vi "Move_Twin_Stacks.vi"(3 "Mode":T5, 5 "Traverse line In":T2 {"Row Duration (mins)" format="%#.1f"; "Row No" min=0; "Trace Gas Concentration (%)" min=0.0 format="%#.2f"; "Emission Rate (l/min)" format="%#.2f"; "Tunnel Speed" format="%#.2f"; "Start X" format="%#.2f"; "Start Y" format="%#.2f"; "Start Z" format="%#.2f"; "End X" format="%#.2f"; "End Y" format="%#.2f"; "End Z" format="%#.2f"; "Averaging time (min)" min=0.0 format="%#.2f"}) -> (0 "Error Message":string, 1 "Status":T1, 2 "Traverse line Out":T2 {"Row Duration (mins)" format="%#.1f"; "Row No" min=0; "Trace Gas Concentration (%)" min=0.0 format="%#.2f"; "Emission Rate (l/min)" format="%#.2f"; "Tunnel Speed" format="%#.2f"; "Start X" format="%#.2f"; "Start Y" format="%#.2f"; "Start Z" format="%#.2f"; "End X" format="%#.2f"; "End Y" format="%#.2f"; "End Z" format="%#.2f"; "Averaging time (min)" min=0.0 format="%#.2f"})   [LabVIEW 2010]
uses:
  Gen Trav/Traverse_cluster.ctl
  Gen Trav/Spacing.ctl
  Controls/Multi_run_mode.ctl
  Controls/User_Specific_mode.ctl
  Gen Trav/Multi_Run_Status.ctl
  ADAM Client/Sub VIs/ADAM Controls/Update_scan_value.ctl
panel:
  out "Delta X":dbl
  out "Trav Position":dbl
  out "Dumb Position":dbl
  # "X           Y            Z"
  # "Start"
  # "End"
  # "X           Y            Z"
  # "Start"
  # "End"
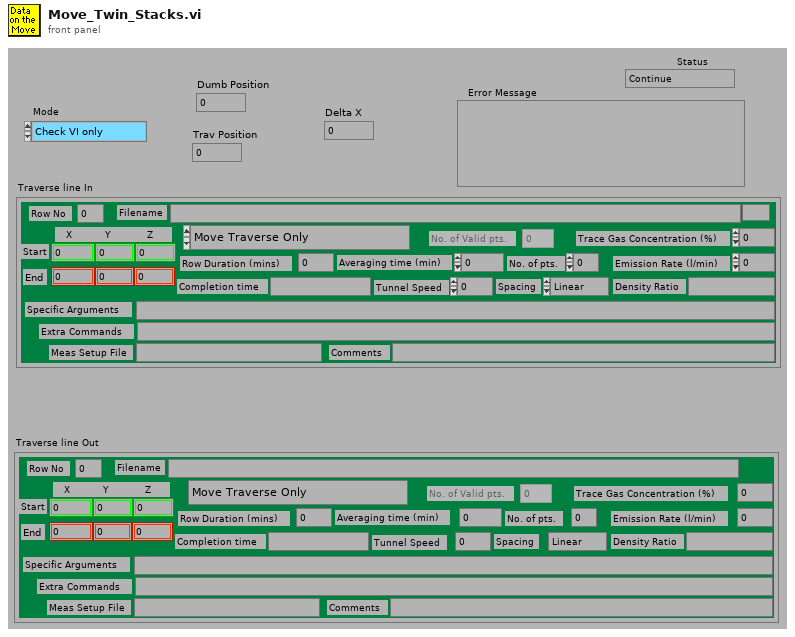
[diagram p1: front panel]
types:
  T1 = typedef "Multi_Run_Status.ctl" = enum16{"Continue", "Jump to Next Point", "Jump to Next Row", "Jump To Fall Back", "Terminate Run"}
  T2 = typedef "Traverse_cluster.ctl" = cluster{"Start X":dbl, "Start Y":dbl, "Start Z":dbl, "End X":dbl, "End Y":dbl, "End Z":dbl, "No. of pts.":i32, "Spacing":T3, "Filename":path, "Tunnel Speed":dbl, "Averaging time (min)":dbl, "Extra Commands":string, "Specific Arguments":string, "Emission Rate (l/min)":dbl, "Trace Gas Concentration (%)":dbl, "Density Ratio":string, "Comments":string, "Row No":i32, "Row Type Selector":T4, "Completion time":string, "Row Duration (mins)":dbl, "No. of Valid pts.":i32, "Meas Setup File":string}
  T3 = typedef "Spacing.ctl" = enum16{"Linear", "Log", "Gauss", "Specified", "N/A"}
  T4 = typedef "Multi_run_mode.ctl" = enum16{"Move Traverse Only", "Set Tunnel Speed Only", "Set Source Only", "Set Measurement Conditions", "Single Measurement", "Vertical Profile", "Lateral Profile", "Longitudinal Profile", "Explore Volume", "Multi-Axis Profile", "Auto Calibrate", "Meas Fast FID Bkgnd", "Check Beam Power", "Scanning Valve Measurement", "Run VI Named:", "Set ADAM Ch", "Wait (minutes)", "Send Message", "Synchronize With:", "Fall Back to this Row", "Turn Off Row Repeating", "Blank Row"}
  T5 = typedef "User_Specific_mode.ctl" = enum16{"Check VI only", "Run VI"}
  T6 = typedef "Update_scan_value.ctl" = cluster{"Channel Name":string, "New Value":dbl}
  T7 = typedef "Status_Cluster.ctl" = cluster{"Status":T1, "Error Type":string, "Error Description":string}
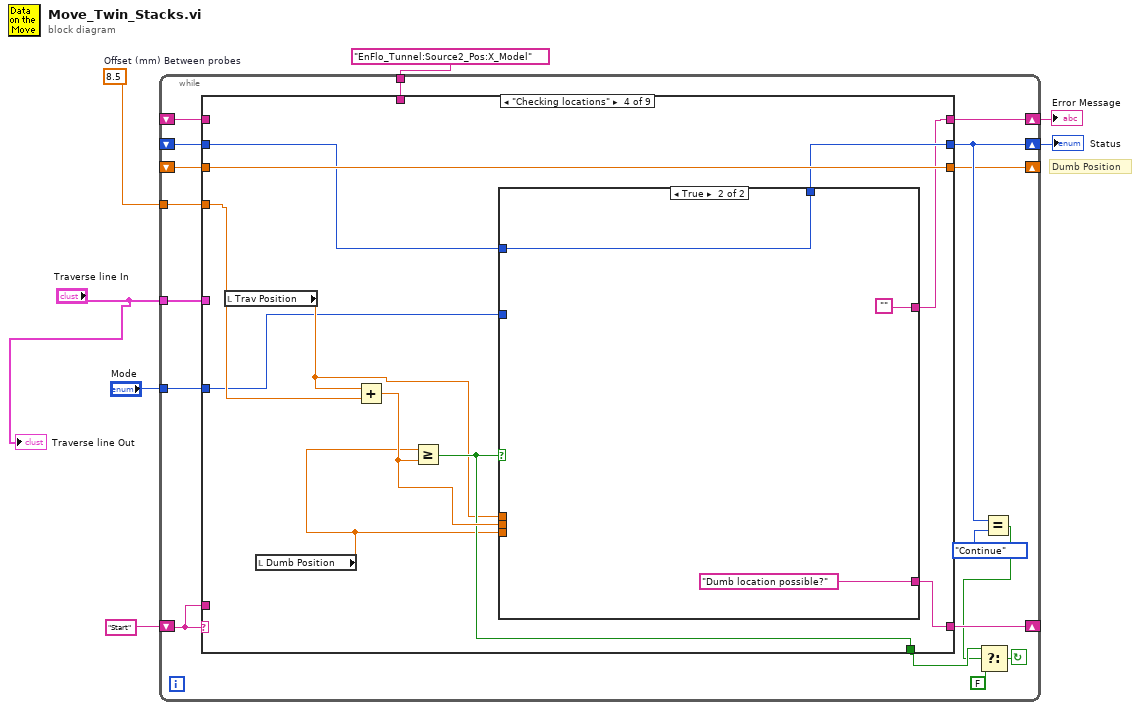
[diagram p0: block diagram]
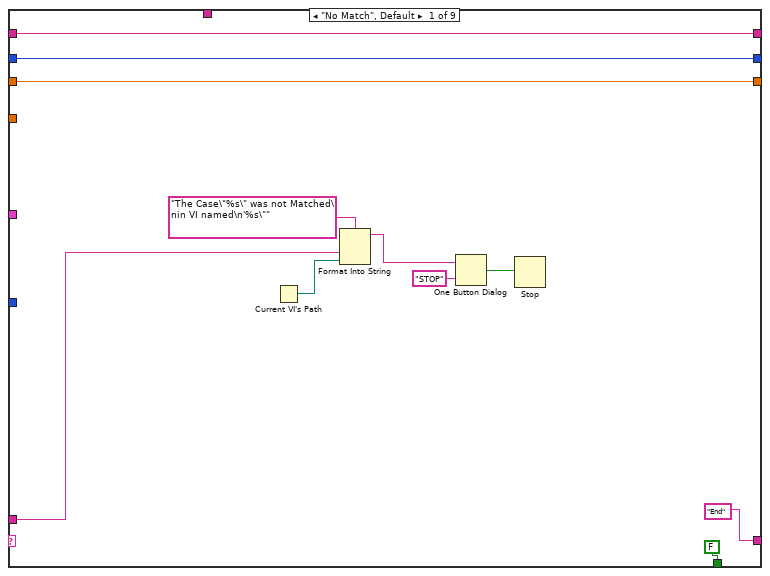
[diagram p2: hidden frame]
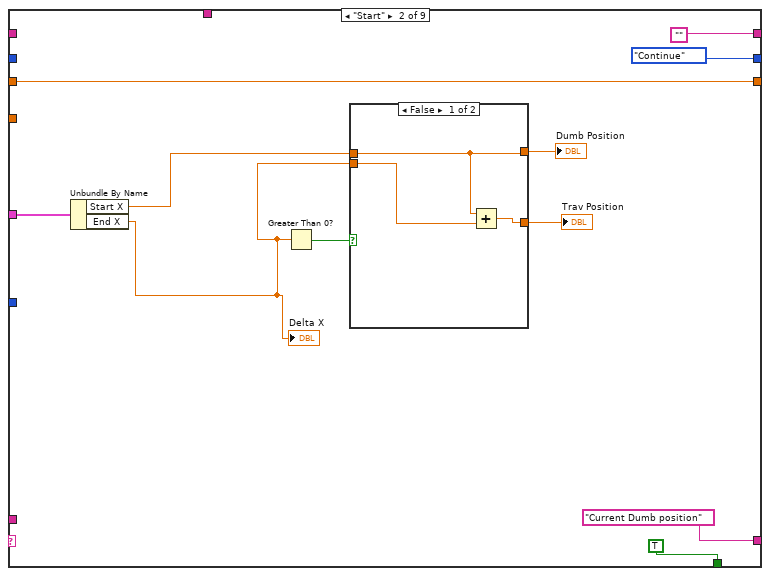
[diagram p3: hidden frame]
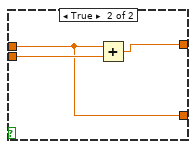
[diagram p4: hidden frame]
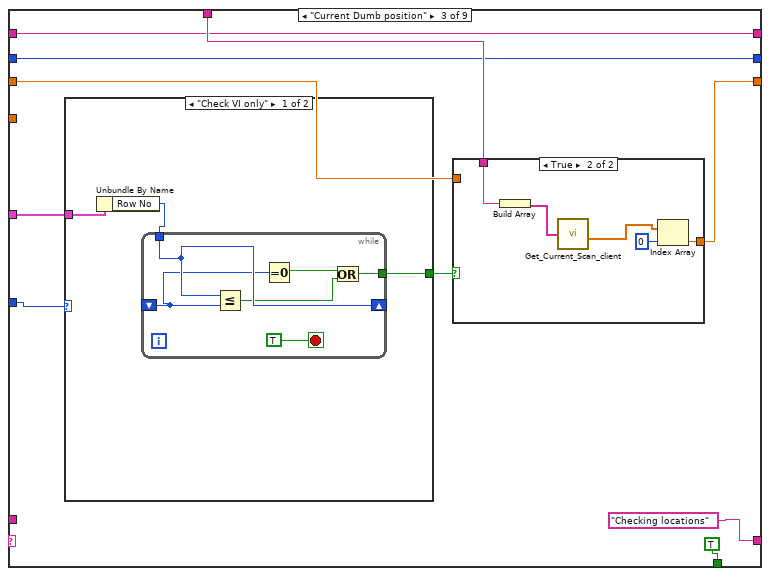
[diagram p5: hidden frame]
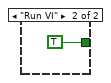
[diagram p6: hidden frame]
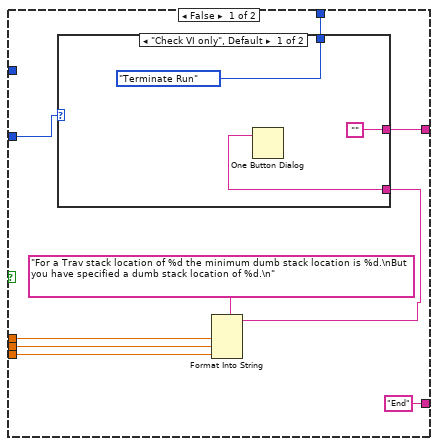
[diagram p8: hidden frame]
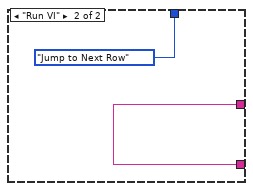
[diagram p9: hidden frame]
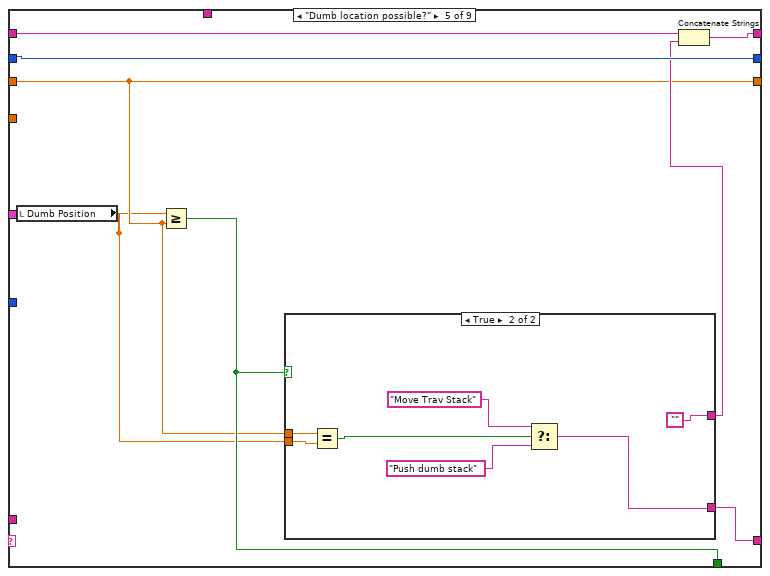
[diagram p10: hidden frame]
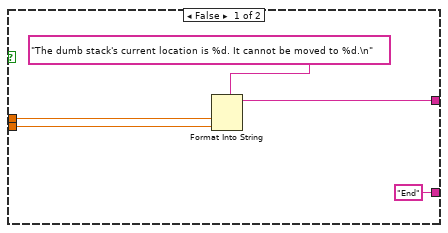
[diagram p11: hidden frame]
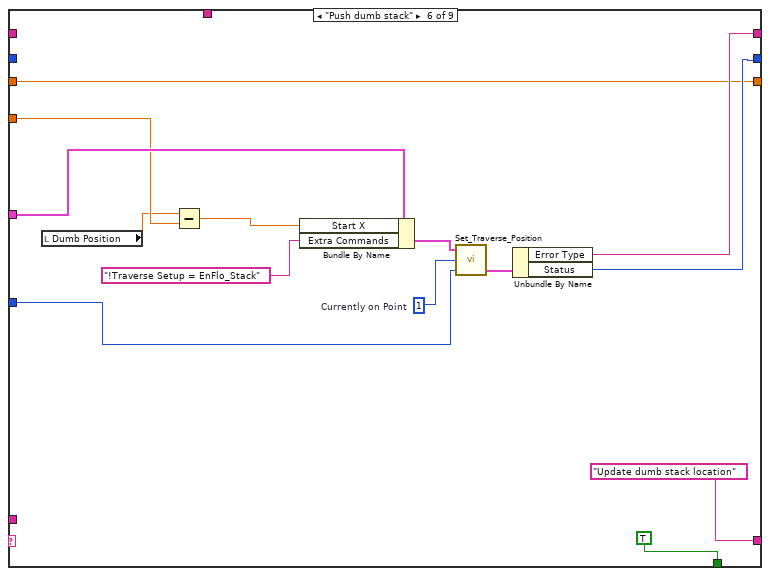
[diagram p12: hidden frame]
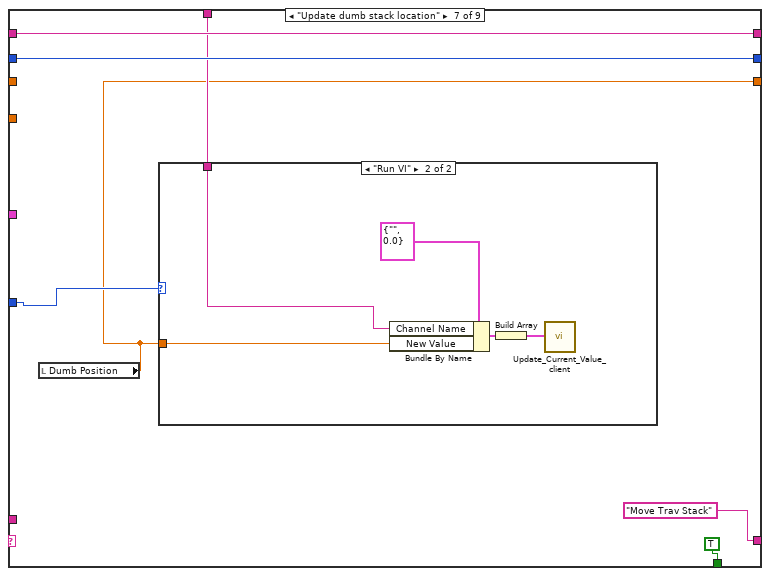
[diagram p13: hidden frame]
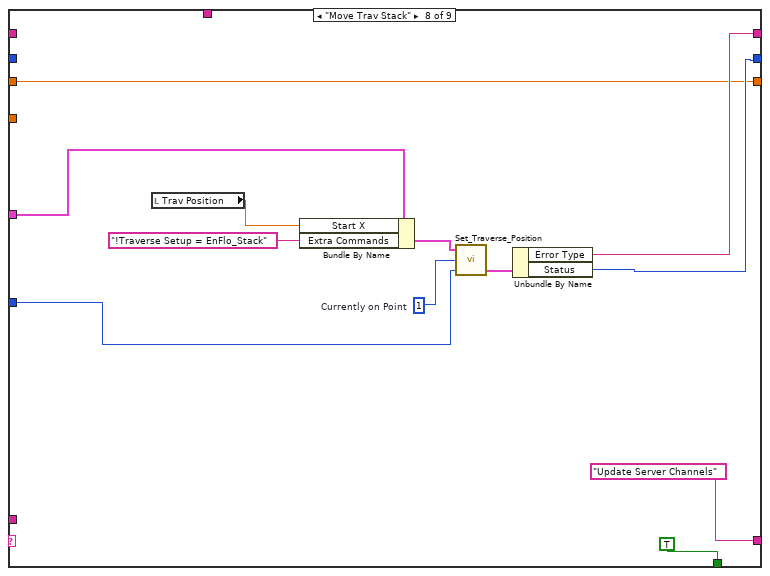
[diagram p15: hidden frame]
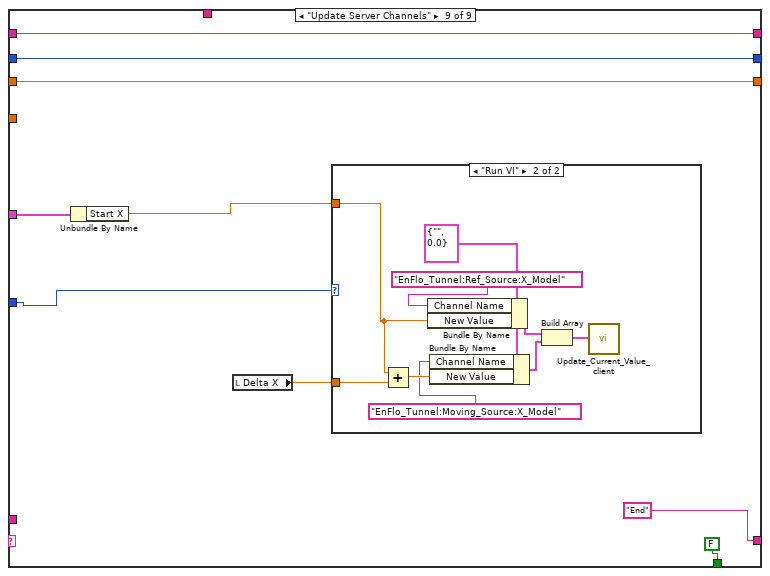
[diagram p16: hidden frame]
diagram:
  w3 = 8.5  # Offset (mm) Between probes
  # "Dumb Position"
  n1 = while {
    shift-left: _ -> [w19]
    shift-right: [w14] -> w4
    shift-left: _ -> [w22]
    shift-right: [w20] -> w5
    tunnel: "Traverse line In" -> [w23]
    tunnel: "Mode" -> [w24]
    shift-left: "Start" -> [w21]
    shift-right: [w18] -> _
    shift-right: [w11] -> _
    shift-left: _ -> [w10]
    tunnel: w3 -> [w9]
    tunnel: "EnFlo_Tunnel:Source2_Pos:X_Model" -> [w8]
    stop <- w12 continue-if-true
    n2 = case shown="\"Checking locations\"" w21 {
      tunnel: w23 -> [_ w46 w53 _ _ w136 _ w159 w168]
      tunnel: w24 -> [_ _ w56 w81 _ w139 w143 w162 w169]
      tunnel: [FALSE ("Update Datum Powers?") TRUE ("Update Datum Powers?") TRUE ("Update Datum Powers?") w87 w113 TRUE ("Update Datum Powers?") TRUE ("Update Datum Powers?") TRUE ("Update Datum Powers?") FALSE ("Update Datum Powers?")] -> w17
      tunnel: ["End" "Current Dumb position" "Checking locations" w86 w108 "Update dumb stack location" "Move Trav Stack" "Update Server Channels" "End"] -> w18
      tunnel: w22 -> [w30 _ w55 _ w110 _ w146 _ w172]
      tunnel: [w30 "" w55 w80 w111 w137 w146 w160 w172] -> w20
      tunnel: w21 -> [w27 _ _ _ _ _ _ _ _]
      tunnel: w19 -> [w26 _ w60 w79 w114 _ w145 _ w171]
      tunnel: [w26 Multi_Run_Status."Continue" ("Status") w60 w82 w114 w130 w145 w156 w171] -> w14
      tunnel: [w25 w39 w62 w83 w109 w129 w141 w154 w166] -> w11
      tunnel: w10 -> [w25 w39 w58 w83 w109 w129 _ w154 w166]
      tunnel: w9 -> [_ _ _ w89 _ w132 _ _ _]
      tunnel: w8 -> [_ _ w61 _ _ _ w142 _ _]
      frame "No Match", Default {
        n3 = Current VI's Path() -> (path=w31:path)
        n4 = Format Into String(format string="The Case\"%s\" was not Matched\nin VI named\n'%s\"" ("Format String"), w27, w31) -> (resulting string=w34:string)  [unwired: 2 in, 1 out]
        n5 = One Button Dialog(message=w34, button name ("OK")="STOP") -> (true=w32:bool)
        n6 = Stop(stop? (T)=w32) -> ()
      }
      frame "Start" {
        n7 = Unbundle By Name(w46) -> ("Start X"=w44:dbl, "End X"=w36:dbl)
        "Delta X" <- w36
        n8 = Greater Than 0?(x=w36) -> (x > 0?=w45:bool)
        n9 = case shown="False" w45 {
          tunnel: w36 -> [w48 w52]
          tunnel: w44 -> [w49 w50]
          tunnel: [w49 w51] -> w43
          tunnel: [w47 w50] -> w42
          frame False {
            n10 = Add(x=w49, y=w48) -> (x+y=w47:dbl)
          }
          frame True {
            n11 = Add(x=w50, y=w52) -> (x+y=w51:dbl)
          }
        }
        "Trav Position" <- w42
        "Dumb Position" <- w43
      }
      frame "Current Dumb position" {
        n12 = case shown="\"Check VI only\"" w56 {
          tunnel: [w65 TRUE] -> w57
          tunnel: w53 -> [w64 _]
          frame "Check VI only" {
            n13 = Unbundle By Name(w64) -> ("Row No"=w63:i32)
            n14 = while {
              shift-right: [w70] -> _
              shift-left: _ -> [w68]
              tunnel: [w66] -> w65
              tunnel: w63 -> [w70]
              stop <- TRUE stop-if-true
              n15 = Less Or Equal?(x=w70, y=w68) -> (x <= y?=w69:bool)
              n16 = Equal To 0?(x=w68) -> (x = 0?=w67:bool)
              n17 = Or(x=w67, y=w69) -> (x .or. y?=w66:bool)
            }
          }
          frame "Run VI" {
          }
        }
        n18 = case shown="True" w57 {
          tunnel: [w73 w74] -> w62
          tunnel: w58 -> [w73 _]
          tunnel: w61 -> [_ w78]
          frame False {
          }
          frame True {
            n19 = Build Array(w78) -> (w77:string[])
            n20 = call "Get_Current_Scan_client.vi"("ADAM Ch Names"=w77) -> ("Numerical Values"=w76:dbl[])  [unwired: 3 out]
            n21 = Index Array(array=w76, index=0) -> (element=w74:dbl)
          }
        }
      }
      frame "Checking locations" {
        n22 = local read "Trav Position"() -> (w84:dbl)
        n23 = local read "Dumb Position"() -> (w85:dbl)
        n24 = Add(x=w84, y=w89) -> (x+y=w88:dbl)
        n25 = Greater Or Equal?(x=w85, y=w88) -> (x >= y?=w87:bool)
        n26 = case shown="True" w87 {
          tunnel: w84 -> [w97 _]
          tunnel: w88 -> [w96 _]
          tunnel: w85 -> [w95 _]
          tunnel: ["End" "Dumb location possible?"] -> w86
          tunnel: [w93 w104] -> w82
          tunnel: w81 -> [w92 _]
          tunnel: [w91 ""] -> w80
          tunnel: w79 -> [_ w104]
          frame False {
            n27 = Format Into String(format string="For a Trav stack location of %d the minimum dumb stack location is %d.\nBut you have specified a dumb stack location of %d.\n", w97, w96, w95) -> (resulting string=w90:string)  [unwired: 2 in, 1 out]
            n28 = case shown="\"Check VI only\", Default" w92 {
              tunnel: [Multi_Run_Status."Terminate Run" ("Status") Multi_Run_Status."Jump to Next Row" ("Status")] -> w93
              tunnel: ["" w103] -> w91
              tunnel: w90 -> [w99 w103]
              frame "Check VI only", Default {
                n29 = One Button Dialog(message=w99) -> ()  [unwired: 2 out]
              }
              frame "Run VI" {
              }
            }
          }
          frame True {
          }
        }
      }
      frame "Dumb location possible?" {
        n30 = local read "Dumb Position"() -> (w107:dbl)
        n31 = Greater Or Equal?(x=w107, y=w109) -> (x >= y?=w113:bool)
        n32 = case shown="True" w113 {
          tunnel: w109 -> [w118 w125]
          tunnel: w107 -> [w117 w124]
          tunnel: [w116 ""] -> w112
          tunnel: ["End" w120] -> w108
          frame False {
            n33 = Format Into String(format string="The dumb stack's current location is %d. It cannot be moved to %d.\n", w118, w117) -> (resulting string=w116:string)  [unwired: 2 in, 1 out]
          }
          frame True {
            n34 = Equal?(x=w125, y=w124) -> (x = y?=w123:bool)
            n35 = Select(t="Move Trav Stack", s=w123, f="Push dumb stack") -> (s? t:f=w120:string)
          }
        }
        n36 = Concatenate Strings(w110, w112) -> (w111:string)
      }
      frame "Push dumb stack" {
        w140 = 1  # Currently on Point
        n37 = local read "Dumb Position"() -> (w127:dbl)
        n38 = Subtract(x=w127, y=w132) -> (x-y=w135:dbl)
        n39 = Bundle By Name(cluster=w136, "Start X"=w135, "Extra Commands"="!Traverse Setup = EnFlo_Stack") -> (w133:T2)
        n40 = call "Set_Traverse_Position.vi"("Simulate/Run"=w139, "Currently on Point"=w140, "Traverse line"=w133) -> ("Status Cluster"=w138:T7)  [unwired: 2 out]
        n41 = Unbundle By Name(w138) -> ("Error Type"=w137:string, "Status"=w130:T1)
      }
      frame "Update dumb stack location" {
        n42 = local read "Dumb Position"() -> (w141:dbl)
        n43 = case shown="\"Run VI\"" w143 {
          tunnel: w141 -> [_ w149]
          tunnel: w142 -> [_ w148]
          frame "Check VI only" {
          }
          frame "Run VI" {
            n44 = Bundle By Name(cluster=T6 {"Channel Name"="", "New Value"=0.0} ("Update Scan Value Cluster"), "Channel Name"=w148, "New Value"=w149) -> (w151:T6)
            n45 = Build Array(w151) -> (w152:T6[])
            n46 = call "Update_Current_Value_client.vi"("Update array in"=w152) -> ()  [unwired: 1 in]
          }
        }
      }
      frame "Move Trav Stack" {
        w163 = 1  # Currently on Point
        n47 = local read "Trav Position"() -> (w153:dbl)
        n48 = Bundle By Name(cluster=w159, "Start X"=w153, "Extra Commands"="!Traverse Setup = EnFlo_Stack") -> (w157:T2)
        n49 = call "Set_Traverse_Position.vi"("Simulate/Run"=w162, "Currently on Point"=w163, "Traverse line"=w157) -> ("Status Cluster"=w161:T7)  [unwired: 2 out]
        n50 = Unbundle By Name(w161) -> ("Error Type"=w160:string, "Status"=w156:T1)
      }
      frame "Update Server Channels" {
        n51 = Unbundle By Name(w168) -> ("Start X"=w167:dbl)
        n52 = local read "Delta X"() -> (w165:dbl)
        n53 = case shown="\"Run VI\"" w169 {
          tunnel: w167 -> [_ w178]
          tunnel: w165 -> [_ w177]
          frame "Check VI only" {
          }
          frame "Run VI" {
            w180 = T6 {"Channel Name"="", "New Value"=0.0} ("Update Scan Value Cluster")
            n54 = Add(x=w178, y=w177) -> (x+y=w176:dbl)
            n55 = Bundle By Name(cluster=w180, "Channel Name"="EnFlo_Tunnel:Ref_Source:X_Model", "New Value"=w178) -> (w181:T6)
            n56 = Bundle By Name(cluster=w180, "Channel Name"="EnFlo_Tunnel:Moving_Source:X_Model", "New Value"=w176) -> (w179:T6)
            n57 = Build Array(w181, w179) -> (w182:T6[])
            n58 = call "Update_Current_Value_client.vi"("Update array in"=w182) -> ()  [unwired: 1 in]
          }
        }
      }
    }
    n59 = Equal?(x=w14, y=Multi_Run_Status."Continue" ("Status")) -> (x = y?=w16:bool)
    n60 = Select(t=w17, s=w16, f=FALSE) -> (s? t:f=w12:bool)
  }
  "Status" <- w4
  "Error Message" <- w5
  "Traverse line Out" <- "Traverse line In"
